vi "Configure Clock Recovery Scale.vi"(4 "Vertical Range (1)":dbl, 6 "Vertical Offset (1)":dbl, 7 "Enable Recovered Clock Display (Enable)":bool, 8 "error in (no error)":errorcluster, 9 "Auto Vertical Scale (Enable)":bool, 10 "Source (1: Channel 1)":i32(ring) items=["Channel 1", "Channel 2", "Channel 3", "Channel 4"], 11 "VISA resource name":refnum<visa-resource-name>) -> (0 "error out":errorcluster, 3 "VISA resource name out":refnum<visa-resource-name>)   [LabVIEW 2009, in "Agilent 8000 Series.lvlib"]
doc: "Enables or disables recovered clock and configures the vertical settings."
uses:
  Agilent 8000 Series.lvlib
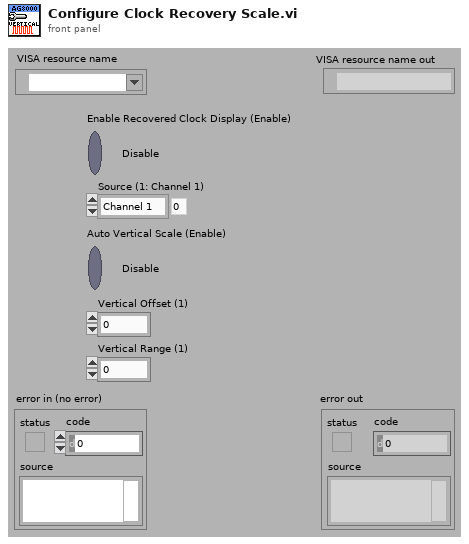
[diagram p1: front panel]
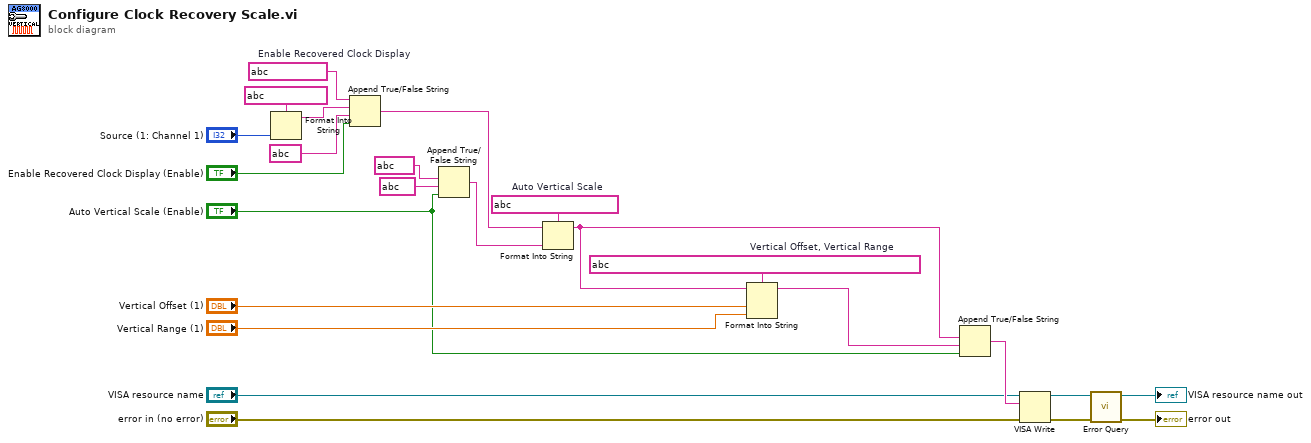
[diagram p0: block diagram]
diagram:
  w14 = string ?  # Auto Vertical Scale
  w18 = string ?  # Enable Recovered Clock Display
  w22 = string ?  # Vertical Offset, Vertical Range
  n1 = Format Into String(format string=string ?, "Source (1: Channel 1)") -> (resulting string=w17:string)  [unwired: 2 in, 1 out]
  n2 = Append True/False String(1:"Enable Recovered Clock Display (Enable)", 2:string ? ("false string"), 3:w17, 4:w18) -> (0:w13:string)
  n3 = Append True/False String(1:"Auto Vertical Scale (Enable)", 2:string ? ("false string"), 3:string ? ("true string")) -> (0:w12:string)  [unwired: 1 in]
  n4 = Format Into String(format string=w14, initial string=w13, w12) -> (resulting string=w9:string)  [unwired: 1 in, 1 out]
  n5 = Format Into String(format string=w22, initial string=w9, "Vertical Offset (1)", "Vertical Range (1)") -> (resulting string=w8:string)  [unwired: 1 in, 1 out]
  n6 = Append True/False String(1:"Auto Vertical Scale (Enable)", 2:w8, 3:w9) -> (0:w7:string)  [unwired: 1 in]
  n7 = VISA Write(VISA resource name="VISA resource name", write buffer=w7, error in (no error)="error in (no error)") -> (VISA resource name out=w4:refnum<visa-resource-name>, error out=w3:errorcluster)  [unwired: 1 out]
  n8 = call "Error Query.vi"("error in (no error)"=w3, "VISA resource name"=w4) -> ("error out"=→"error out":errorcluster, "VISA resource name out"=→"VISA resource name out":refnum<visa-resource-name>)  [unwired: 6 in, 2 out]
